vi "Write dFrequencyVoltageRange.vi"(8 "error in (no error)":errorcluster, 10 "dFrequencyVoltageRange":dbl, 11 "NISTSamplerPluginsBase in":refnum<class "SamplerPluginsBase.lvclass">) -> (0 "error out":errorcluster, 3 "NISTSamplerPluginsBase out":refnum<class "SamplerPluginsBase.lvclass">)   [LabVIEW 2014, in "SamplerPlugins.lvlib" / "SamplerPluginsBase.lvclass"]
uses:
  SamplerPluginsBase.lvclass
  SamplerPluginsBase.lvclass/SamplerPluginsBase.ctl
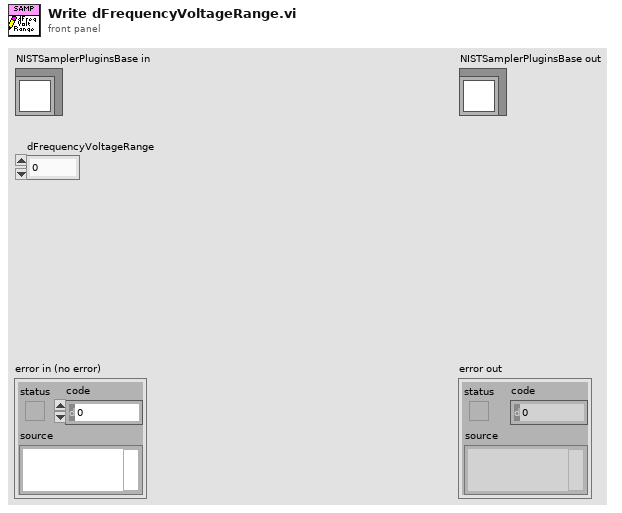
[diagram p1: front panel]
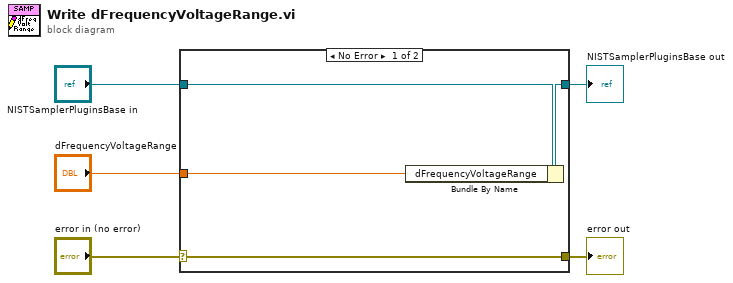
[diagram p0: block diagram]
diagram:
  n1 = case shown="No Error" "error in (no error)" {
    selector: "error in (no error)" -> [w9 w10]
    tunnel: [w9 w10] -> w4
    tunnel: [w7 w11] -> w2
    tunnel: "NISTSamplerPluginsBase in" -> [w8 w11]
    tunnel: "dFrequencyVoltageRange" -> [w6 _]
    frame No Error {
      n2 = Bundle By Name(cluster=w8, "dFrequencyVoltageRange"=w6) -> (w7:refnum<class "SamplerPluginsBase.lvclass">)
    }
    frame Error {
    }
  }
  "error out" <- w4
  "NISTSamplerPluginsBase out" <- w2
